vi "Maui.Test.DefaultDirectory.RunAllTests.vi"(8 "error in (no error)":errorcluster, 11 "TestDefaultDirectory in":refnum<class "Maui.Test.DefaultDirectory.lvclass">) -> (0 "error out":errorcluster, 3 "TestDefaultDirectory out":refnum<class "Maui.Test.DefaultDirectory.lvclass">)   [LabVIEW 2020, in "Maui.Test.DefaultDirectory.lvclass"]
uses:
  Maui.Test.DefaultDirectory.lvclass
  <vilib>/addons/_JKI Toolkits/Caraya/classes/Test/Test.lvclass
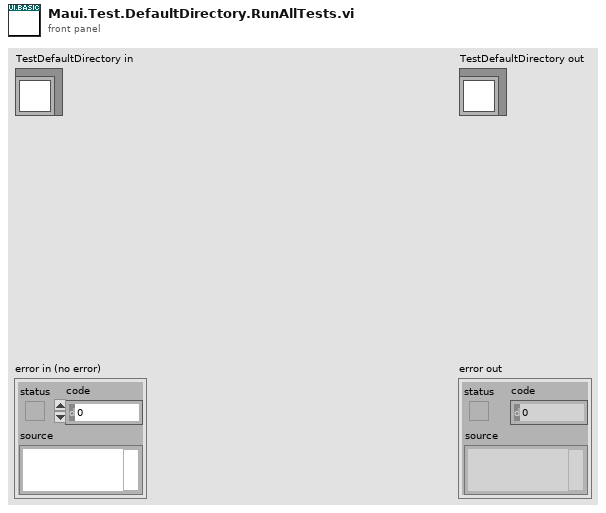
[diagram p1: front panel]
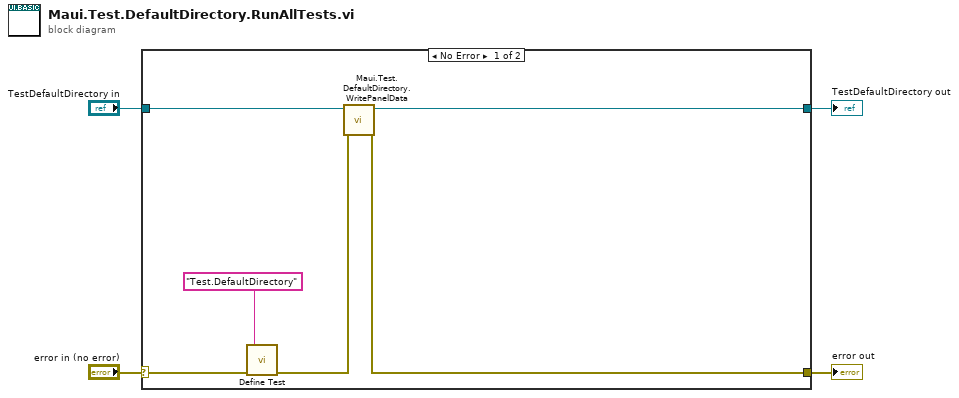
[diagram p0: block diagram]
diagram:
  n1 = case shown="No Error" "error in (no error)" {
    selector: "error in (no error)" -> [w10 w12]
    tunnel: [w7 w12] -> w3
    tunnel: [w6 w11] -> w1
    tunnel: "TestDefaultDirectory in" -> [w5 w11]
    frame No Error {
      n2 = call <vilib>:"Define Test.vi"("error in (no error)"=w10, "Label (VI Title)"="Test.DefaultDirectory") -> ("error out"=w8:errorcluster)  [unwired: 9 in]
      n3 = call "Maui.Test.DefaultDirectory.WritePanelData.vi"("error in (no error)"=w8, "Maui.Test.DefaultDirectory in"=w5) -> ("error out"=w7:errorcluster, "Maui.Test.DefaultDirectory out"=w6:refnum<class "Maui.Test.DefaultDirectory.lvclass">)  [unwired: 8 in]
    }
    frame Error {
    }
  }
  "error out" <- w3
  "TestDefaultDirectory out" <- w1
